vi "rotate colors.vi"(11 "Color Array":u32[](array[colorbox])=[16711680, 16448250, 16860, 6618880, 29469, 16762457, 9282, 13108736, 16765970, 29695, 15689728, 1149184, 5881343, 7536657]) -> (3 "new picture":picture)   [LabVIEW 2015]
panel:
  in  "Zoom Factor":sgl(slide) scale=0.0..10.0
  out "Numeric":i32
  in  "milliseconds to wait":u32(slide) scale=0.0..1000.0
  in  "stop":bool
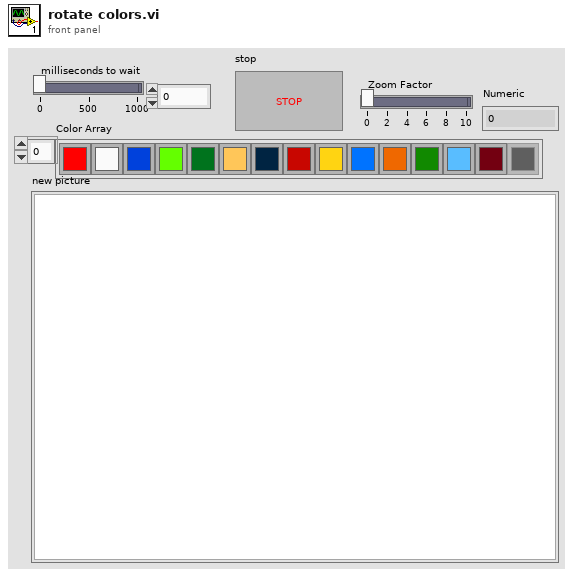
[diagram p1: front panel]
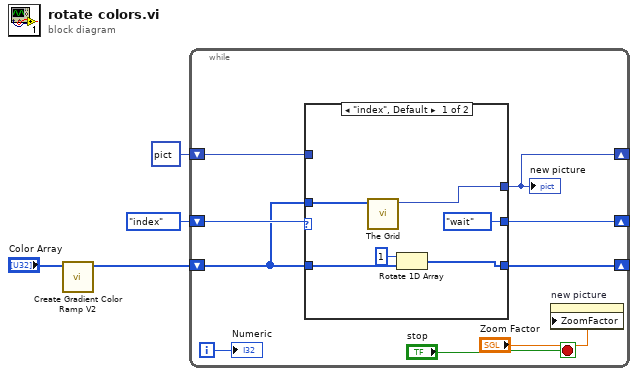
[diagram p0: block diagram]
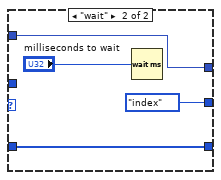
[diagram p2: hidden frame]
diagram:
  n1 = call "Create Gradient Color Ramp V2.vi"("Color Array"="Color Array") -> ("Color Table"=w3:u32[])  [unwired: 8 in, 2 out]
  n2 = while {
    shift-right: [w11] -> _
    shift-left: enum16{"index", "wait"}."index" -> [w12]
    shift-right: [w5] -> _
    shift-left: picture data[5B] ("new picture") -> [w10]
    shift-right: [w9] -> _
    shift-left: w3 -> [w8]
    i -> [w7]
    stop <- "stop" stop-if-true
    n3 = case shown="\"index\", Default" w12 {
      tunnel: w8 -> [w19 _]
      tunnel: [enum16{"index", "wait"}."wait" enum16{"index", "wait"}."index"] -> w11
      tunnel: [w17 w21] -> w5
      tunnel: w10 -> [_ w21]
      tunnel: [w15 w20] -> w9
      tunnel: w8 -> [w16 w20]
      frame "index", Default {
        n4 = call "The Grid.vi"("Color Array"=w19) -> ("new picture"=w17:picture)  [unwired: 10 in]
        n5 = Rotate 1D Array(1:w16, 2:1 ("n")) -> (0:w15:u32[])
      }
      frame "wait" {
        n6 = Wait (ms)(milliseconds to wait="milliseconds to wait") -> ()  [unwired: 1 out]
      }
    }
    "new picture" <- w5
    n7 = property on="new picture" class="Pict"("ZoomFactor"="Zoom Factor") -> ()  [unwired: 2 in, 2 out]
    "Numeric" <- w7
  }
